vi "SetText__slk_mt.vi"(8 "error in (no error)":errorcluster, 10 "text":string, 11 "label in":refnum<class "Label__slk_mt.lvclass">) -> (0 "error out":errorcluster, 3 "label out":refnum<class "Label__slk_mt.lvclass">)   [LabVIEW 2012, in "Lazyboots Menu Tool.lvlib" / "Label__slk_mt.lvclass"]
doc: "Sets text of label object."
uses:
  Label__slk_mt.lvclass
panel:
  # "SetText__slk_mt.vi\nSets text of label object.\n\nNOTICE -- YOU MUST LEAVE THIS NOTICE IN PLACE.\n\nCopyright (c) 2011, LIANG LIU Shawn.Liu.cn@gmail.com\nAll rights reserved.\n\nRedistribution and use in source and binary forms, with or without modification, are permitted provided that the following conditions are met:\n-Redistributions of source code must retain the above copyright notice, this list of conditions and the following disclaimer.\n-Redistributions in binary form must reproduce the above copyright notice, this list of conditions and the following disclaimer in the documentation and/or other materials provided with the distribution.\n-Neither the name of the eLp nor the names of its contributors may be used to endorse or promote products derived from this software without specific prior written permission.\n\nTHIS SOFTWARE IS PROVIDED BY THE COPYRIGHT HOLDERS AND CONTRIBUTORS \"AS IS\" AND ANY EXPRESS OR IMPLIED WARRANTIES, INCLUDING, BUT NOT LIMITED TO, THE IMPLIED WARRANTIES OF MERCHANTABILITY AND FITNESS FOR A PARTICULAR PURPOSE ARE DISCLAIMED. IN NO EVENT SHALL THE COPYRIGHT HOLDER OR CONTRIBUTORS BE LIABLE FOR ANY DIRECT, INDIRECT, INCIDENTAL, SPECIAL, EXEMPLARY, OR CONSEQUENTIAL DAMAGES (INCLUDING, BUT NOT LIMITED TO, PROCUREMENT OF SUBSTITUTE GOODS OR SERVICES; LOSS OF USE, DATA, OR PROFITS; OR BUSINESS INTERRUPTION) HOWEVER CAUSED AND ON ANY THEORY OF LIABILITY, WHETHER IN CONTRACT, STRICT LIABILITY, OR TORT (INCLUDING NEGLIGENCE OR OTHERWISE) ARISING IN ANY WAY OUT OF THE USE OF THIS SOFTWARE, EVEN IF ADVISED OF THE POSSIBILITY OF SUCH DAMAGE."
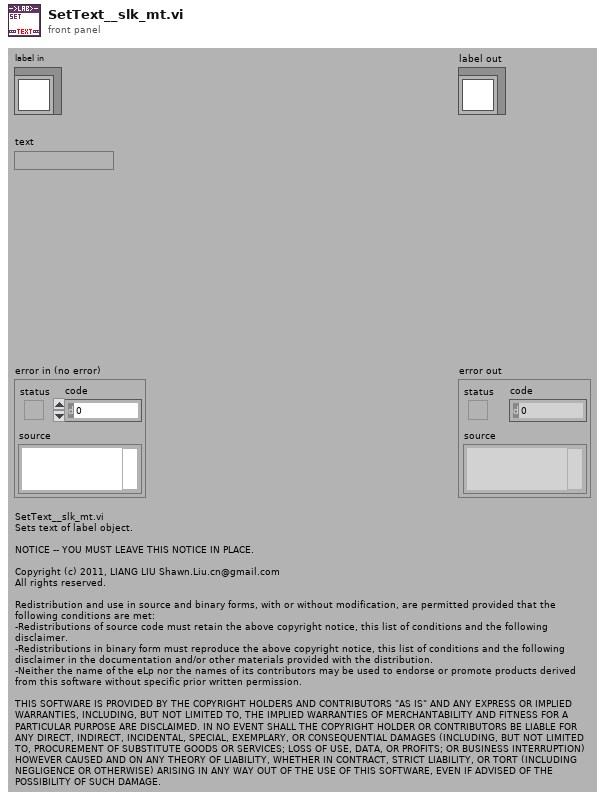
[diagram p1: front panel]
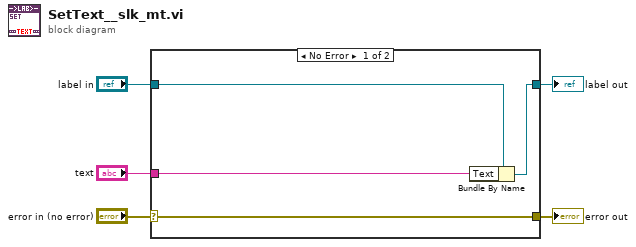
[diagram p0: block diagram]
diagram:
  n1 = case shown="No Error" "error in (no error)" {
    selector: "error in (no error)" -> [w6 w10]
    tunnel: [w6 w10] -> w4
    tunnel: [w8 w11] -> w2
    tunnel: "label in" -> [w9 w11]
    tunnel: "text" -> [w7 _]
    frame No Error {
      n2 = Bundle By Name(cluster=w9, "Text"=w7) -> (w8:refnum<class "Label__slk_mt.lvclass">)
    }
    frame Error {
    }
  }
  "error out" <- w4
  "label out" <- w2
